vi "oa_Check Waveform (N Channels).vi"(8 "error in (no error)":errorcluster, 11 "scaled signal":waveform(dbl)[](array[waveform])) -> (0 "error out":errorcluster, 1 "empty signal":bool, 3 "scaled signal out":waveform(dbl)[](array[waveform]))   [LabVIEW 2017, in "SoundVib_Resampling.lvlib"]
uses:
  <vilib>/addons/Sound and Vibration/Order Analysis/Resample Order Tracking/SoundVib_Resampling.lvlib
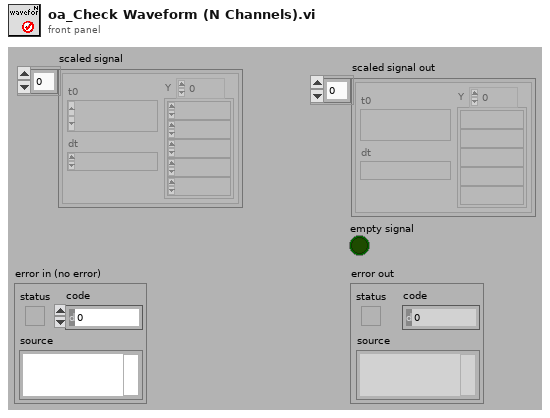
[diagram p1: front panel]
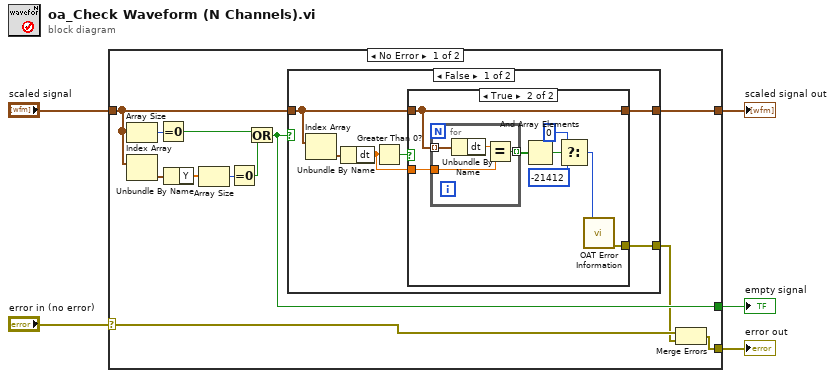
[diagram p0: block diagram]
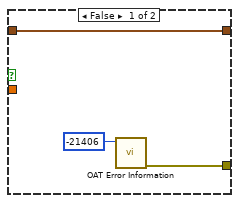
[diagram p2: hidden frame]
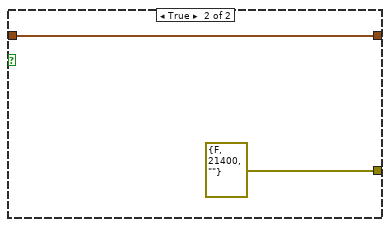
[diagram p3: hidden frame]
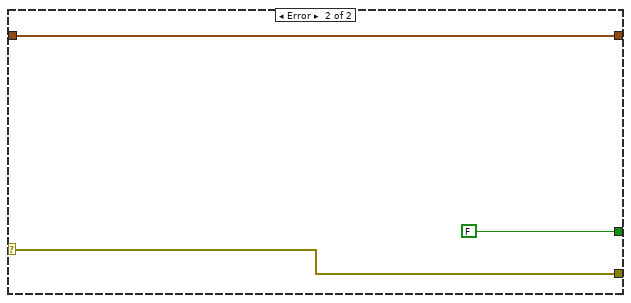
[diagram p4: hidden frame]
diagram:
  n1 = case shown="No Error" "error in (no error)" {
    selector: "error in (no error)" -> [w8 w43]
    tunnel: "scaled signal" -> [w10 w42]
    tunnel: [w6 w43] -> w3
    tunnel: [w11 FALSE] -> w2
    tunnel: [w9 w42] -> w1
    frame No Error {
      n2 = Array Size(array=w10) -> (size(s)=w17:i32)
      n3 = Index Array(array=w10) -> (element=w16:waveform(dbl))  [unwired: 1 in]
      n4 = Equal To 0?(x=w17) -> (x = 0?=w13:bool)
      n5 = Unbundle By Name(w16) -> ("Y"=w14:dbl[])
      n6 = Array Size(array=w14) -> (size(s)=w15:i32)
      n7 = Equal To 0?(x=w15) -> (x = 0?=w12:bool)
      n8 = Or(x=w13, y=w12) -> (x .or. y?=w11:bool)
      n9 = case shown="False" w11 {
        tunnel: [w19 errorcluster {"status"=FALSE, "code"=21400, "source"=""} ("error IO")] -> w7
        tunnel: w10 -> [w22 w39]
        tunnel: [w20 w39] -> w9
        frame False {
          n10 = Index Array(array=w22) -> (element=w23:waveform(dbl))  [unwired: 1 in]
          n11 = Unbundle By Name(w23) -> ("dt"=w18:dbl)
          n12 = Greater Than 0?(x=w18) -> (x > 0?=w21:bool)
          n13 = case shown="True" w21 {
            tunnel: w22 -> [w26 w34]
            tunnel: [w26 w34] -> w20
            tunnel: [w24 w27] -> w19
            tunnel: w18 -> [_ w33]
            frame False {
              n14 = call <vilib>:"OAT Error Information.vi"("error code"=-21406 ("code")) -> ("error out"=w24:errorcluster)  [unwired: 6 in]
            }
            frame True {
              n15 = for {
                tunnel: w34 -> [w38] mode=indexing
                tunnel: w33 -> [w36]
                tunnel: [w35] -> w32 mode=indexing
                n16 = Unbundle By Name(w38) -> ("dt"=w37:dbl)
                n17 = Equal?(x=w37, y=w36) -> (x = y?=w35:bool)
              }
              n18 = And Array Elements(Boolean array=w32) -> (logical AND=w31:bool)
              n19 = Select(t=0 ("code"), s=w31, f=-21412 ("code")) -> (s? t:f=w29:i32)
              n20 = call <vilib>:"OAT Error Information.vi"("error code"=w29) -> ("error out"=w27:errorcluster)  [unwired: 6 in]
            }
          }
        }
        frame True {
        }
      }
      n21 = Merge Errors(w8, w7) -> (w6:errorcluster)
    }
    frame Error {
    }
  }
  "error out" <- w3
  "scaled signal out" <- w1
  "empty signal" <- w2
